vi "ManualControlL0NOGENASICTEST.vi"() -> ()   [LabVIEW 2012]
uses:
  <vilib>/Utility/NIReport.llb/NI_report.lvclass
  <vilib>/Utility/NIReport.llb/HTML/NI_HTML.lvclass
panel:
  in  "Sum/Maj":bool=TRUE
  in  "Ib Clip select":i32(slide)=63 scale=0.0..63.0
  in  "Clipping Select":i32(slide)=1 scale=1.0..3.0
  in  "Attenuation Select":i32(slide) scale=0.0..15.0
  in  "Channel Enable":i32(slide) scale=0.0..6.0
  in  "stop":bool
  in  "Instrument VISA in":T1={"AWG VISA"="AgilentGenerator1", "Oscilloscope  VISA "="AgilentOsciloscope", "Integration Board IP"="172.16.17.47", "connection ID"=refnum, "report out"=refnum, "report file path"=path "C:/Documents and Settings/CTA_LAB01/Desktop/L0_Asic/L0 Asic Test Data"}
  out "error out":errorcluster
  in  "error in":errorcluster
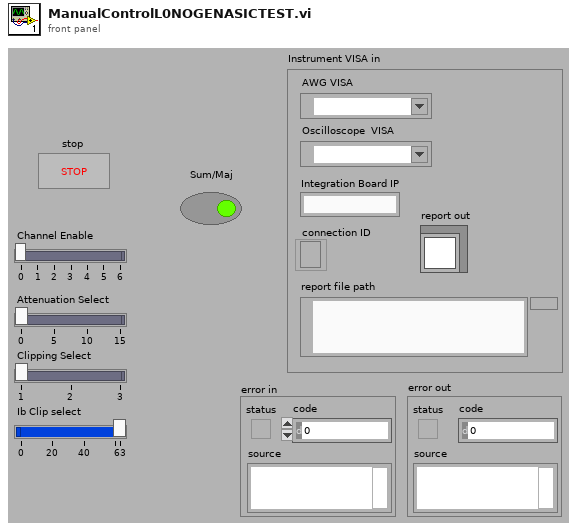
[diagram p1: front panel]
types:
  T1 = cluster{"AWG VISA":refnum<visa-resource-name>, "Oscilloscope  VISA ":refnum<visa-resource-name>, "Integration Board IP":string, "connection ID":refnum<k5>, "report out":refnum<class "NI_report.lvclass">, "report file path":path}
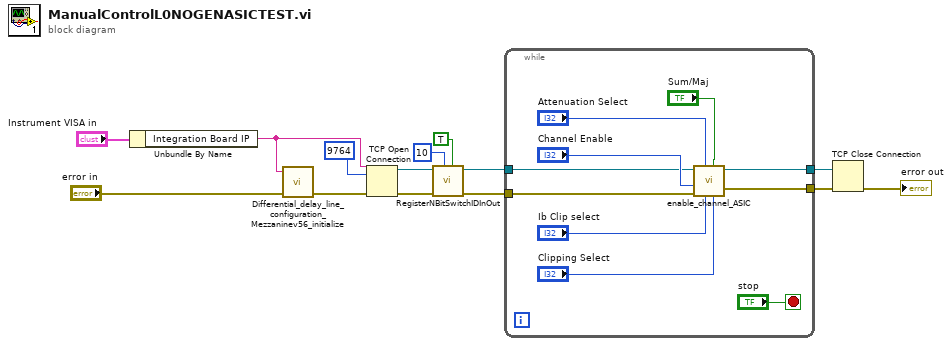
[diagram p0: block diagram]
diagram:
  n1 = Unbundle By Name("Instrument VISA in") -> ("Integration Board IP"=w2:string)
  n2 = call "Differential_delay_line_configuration_Mezzaninev56_initialize.vi"("error in (no error)"="error in", "address"=w2) -> ("error out 2"=w11:errorcluster)  [unwired: 1 in]
  n3 = TCP Open Connection(address=w2, remote port or service name=9764, error in (no error)=w11) -> (connection ID=w6:refnum<k5>, error out=w10:errorcluster)  [unwired: 2 in]
  n4 = call "RegisterNBitSwitchIDInOut.vi"("Switch Bit"=TRUE, "N Bit"=10, "error in (no error)"=w10, "connection ID"=w6) -> ("error out"=w7:errorcluster, "connection ID out"=w5:refnum<k5>)  [unwired: 5 in]
  n5 = while {
    tunnel: [w18] -> w9
    tunnel: [w17] -> w8
    tunnel: w7 -> [w20]
    tunnel: w5 -> [w19]
    stop <- "stop" stop-if-true
    n6 = call "enable_channel_ASIC.vi"("Clip_sel_b"="Clipping Select", "maj/sum"="Sum/Maj", "Ib_clipVb"="Ib Clip select", "Att gain"="Attenuation Select", "error in"=w20, "Channel"="Channel Enable", "connection ID"=w19) -> ("error out"=w18:errorcluster, "connection ID out"=w17:refnum<k5>)  [unwired: 2 in, 1 out]
  }
  n7 = TCP Close Connection(connection ID=w8, error in (no error)=w9) -> (error out=→"error out":errorcluster)  [unwired: 1 in, 1 out]
